vi "Configure External Data Log.vi"(5 "External Data Log Period (0.1 s)":dbl=0.1, 6 "Enable Minimum Maximum Log (False)":bool, 7 "Enable External Data Log (False)":bool, 8 "error in (no error)":errorcluster {"code" format="%.0x"}, 9 "External Data Log Type (1: Voltage)":i32(ring)=1 items=["Voltage"=1, "Current"=0], 10 "Channel Name (1)":string="1", 11 "VISA resource name":refnum<visa-resource-name>) -> (0 "error out":errorcluster {"code" format="%.0x"}, 3 "VISA resource name out":refnum<visa-resource-name>)   [LabVIEW 2010, in "Agilent N6700 Series.lvlib"]
doc: "Configures the external data log."
uses:
  Agilent N6700 Series.lvlib
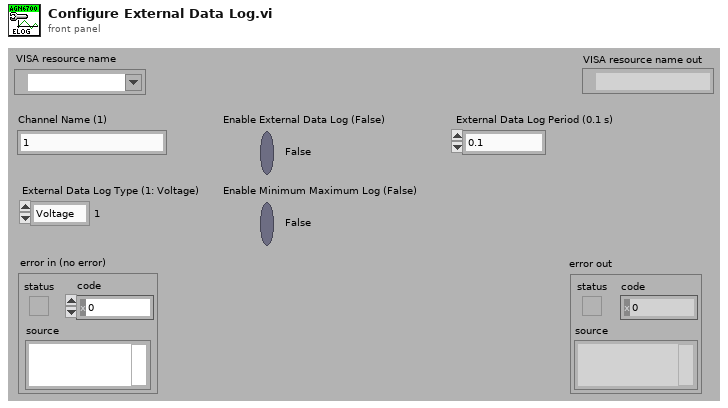
[diagram p1: front panel]
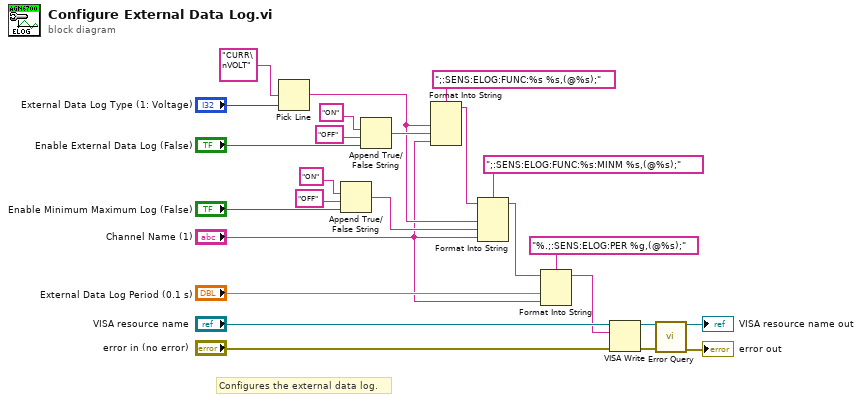
[diagram p0: block diagram]
diagram:
  # "Configures the external data log."
  n1 = Pick Line(multi-line string="CURR\nVOLT", line index="External Data Log Type (1: Voltage)") -> (output string=w5:string)  [unwired: 1 in]
  n2 = Append True/False String(1:"Enable Minimum Maximum Log (False)", 2:"OFF", 3:"ON") -> (0:w4:string)  [unwired: 1 in]
  n3 = Append True/False String(1:"Enable External Data Log (False)", 2:"OFF", 3:"ON") -> (0:w12:string)  [unwired: 1 in]
  n4 = Format Into String(format string=";:SENS:ELOG:FUNC:%s %s,(@%s);", w5, w12, "Channel Name (1)") -> (resulting string=w1:string)  [unwired: 2 in, 1 out]
  n5 = Format Into String(format string=";:SENS:ELOG:FUNC:%s:MINM %s,(@%s);", initial string=w1, w5, w4, "Channel Name (1)") -> (resulting string=w3:string)  [unwired: 1 in, 1 out]
  n6 = Format Into String(format string="%.;:SENS:ELOG:PER %g,(@%s);", initial string=w3, "External Data Log Period (0.1 s)", "Channel Name (1)") -> (resulting string=w10:string)  [unwired: 1 in, 1 out]
  n7 = VISA Write(VISA resource name="VISA resource name", write buffer=w10, error in (no error)="error in (no error)") -> (VISA resource name out=w21:refnum<visa-resource-name>, error out=w20:errorcluster)  [unwired: 1 out]
  n8 = call "Error Query.vi"("VISA resource name"=w21, "error in (no error)"=w20) -> ("VISA resource name out"=→"VISA resource name out":refnum<visa-resource-name>, "error out"=→"error out":errorcluster)  [unwired: 10 in, 2 out]
